vi "FPGA ADC IO Node_Core.vi"(9 "input valid (nc)":bool=TRUE, 11 "rx core":refnum<class "niUSRP Rx Core v1 FPGA.lvclass">, 12 "ready for output (t)":bool=TRUE, 13 "trigger":bool) -> (4 "data":T1[](array[typedef]), 10 "output valid":bool, 14 "ready for input (nc)":bool, 15 "rx core":refnum<class "niUSRP Rx Core v1 FPGA.lvclass">)   [LabVIEW 2025, in "niUSRP Rx Core v1 FPGA.lvclass"]
uses:
  niUSRP Rx Core v1 FPGA.lvclass
  <instrlib>/_niInstr/DSP/v1/Shared/Public/IQ Data.ctl
  <instrlib>/_niInstr/DSP/v1/Shared/niInstr DSP v1 Shared.lvlib
  <instrlib>/_niInstr/Basic Elements/v1/FPGA/niInstr Basic Elements v1 FPGA.lvlib
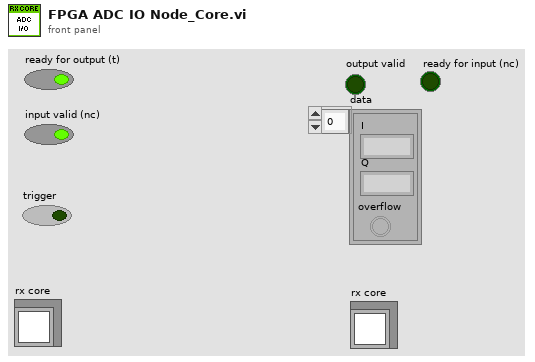
[diagram p1: front panel]
types:
  T1 = typedef "niInstr DSP v1 Shared.lvlib/IQ Data.ctl" = cluster{"I":fxp<+/-,18,1>, "Q":fxp<+/-,18,1>, "overflow":bool}
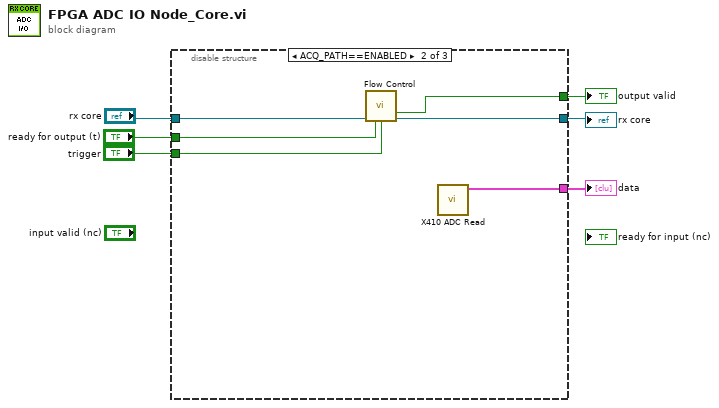
[diagram p0: block diagram]
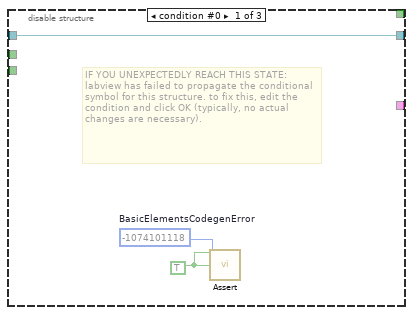
[diagram p2: hidden frame]
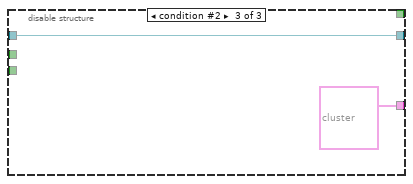
[diagram p3: hidden frame]
diagram:
  n1 = disable-structure shown="ACQ_PATH==ENABLED" {
    disable-tunnel: "rx core" -> [w7 w11 w16]
    disable-tunnel: [_ w15 T1[] [{"I"=0.0, "Q"=0.0, "overflow"=FALSE}, {"I"=0.0, "Q"=0.0, "overflow"=FALSE}, {"I"=0.0, "Q"=0.0, "overflow"=FALSE}, {"I"=0.0, "Q"=0.0, "overflow"=FALSE}, {"I"=0.0, "Q"=0.0, "overflow"=FALSE}, {"I"=0.0, "Q"=0.0, "overflow"=FALSE}, {"I"=0.0, "Q"=0.0, "overflow"=FALSE}, {"I"=0.0, "Q"=0.0, "overflow"=FALSE}] ("IQ Data")] -> w6
    disable-tunnel: [w7 w10 w16] -> w4
    disable-tunnel: [_ w14 _] -> w3
    disable-tunnel: "ready for output (t)" -> [_ w13 _]
    disable-tunnel: "trigger" -> [_ w12 _]
    frame condition #0 {
      w9 = TRUE ("assert")
      w8 = -1074101118  # BasicElementsCodegenError
      # "IF YOU UNEXPECTEDLY REACH THIS STATE:\nlabview has failed to propagate the conditional symbol for this structure. to fix this, edit the condition and click OK (typically, no actual changes are necessary)."
      n2 = call <instrlib>:"Assert.vi"("assert"=w9, "error code"=w8, "enable show error"=w9) -> ()  [unwired: 13 in]
    }
    frame condition #1 (active) {
      n3 = call-dynamic "Flow Control.vi"("rx core"=w11, "ready for output (t)"=w13, "trigger"=w12) -> ("output valid"=w14:bool, "rx core"=w10:refnum<class "niUSRP Rx Core v1 FPGA.lvclass">)  [unwired: 10 in, 1 out]
      n4 = call "X410 ADC Read.vi"() -> ("Data out"=w15:T1[])  [unwired: 11 in]
    }
    frame condition #2 {
    }
  }
  "data" <- w6
  "rx core" <- w4
  "output valid" <- w3
